vi "6612-00.vi"(8 "error in":errorcluster caption="错误输入") -> (0 "error out":errorcluster caption="错误输出", 3 "task out":refnum<k21> caption="任务输出")   [LabVIEW 2020]
uses:
  <vilib>/DAQmx/create/channels.llb/DAQmx Create Channel (CI-Position-Angular Encoder).vi
  <resource>/objmgr/daqmx.rc
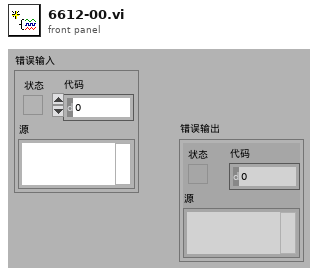
[diagram p1: front panel]
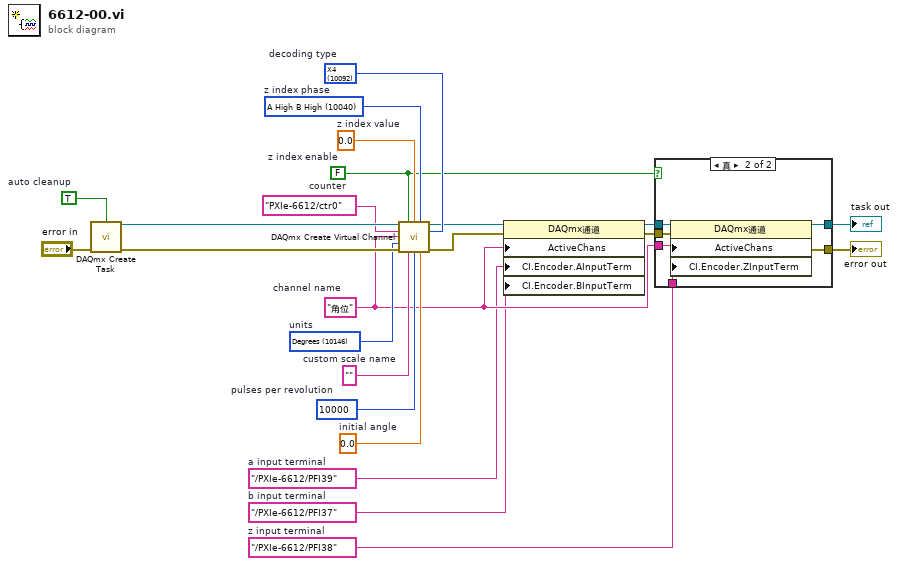
[diagram p0: block diagram]
diagram:
  w1 = "/PXIe-6612/PFI38"  # z input terminal
  w2 = "/PXIe-6612/PFI37"  # b input terminal
  w3 = "/PXIe-6612/PFI39"  # a input terminal
  w15 = 10146 items=["Degrees"=10146, "Radians"=10273, "Ticks"=10304, "From Custom Scale"=10065]  # units
  w11 = 10092 items=["X1"=10090, "X2"=10091, "X4"=10092, "Two Pulse Counting"=10313]  # decoding type
  w12 = 0.0  # initial angle
  w13 = u32 10000  # pulses per revolution
  w14 = ""  # custom scale name
  w16 = 10040 items=["A High B High"=10040, "A High B Low"=10041, "A Low B High"=10042, "A Low B Low"=10043]  # z index phase
  w17 = 0.0  # z index value
  w5 = FALSE  # z index enable
  w4 = "角位"  # channel name
  w19 = "PXIe-6612/ctr0"  # counter
  w21 = TRUE  # auto cleanup
  n1 = call <vilib>:"DAQmx Create Task.vi"("auto cleanup"=w21, "error in"="error in") -> ("task out"=w20:refnum<k21>, "error out"=w22:errorcluster)  [unwired: 12 in]
  n2 = call-poly <vilib>:"DAQmx Create Virtual Channel.vi"("task in"=w20, "z index enable"=w5, "z index value"=w17, "z index phase"=w16, "counter"=w19, "decoding type"=w11, "name to assign"=w4, "units"=w15, "error in"=w22, "custom scale name"=w14, "pulses per revolution"=w13, "initial angle"=w12) -> ("task out"=w10:refnum<k21>, "error out"=w18:errorcluster)  [unwired: 2 in]
  n3 = property class="DAQmx通道"(reference=w10, error in=w18, "ActiveChans"=w4, "CI.Encoder.AInputTerm"=w3, "CI.Encoder.BInputTerm"=w2) -> (reference out=w9:refnum<k21>, error out=w8:errorcluster)
  n4 = case "条件结构" shown="真" w5 {
    tunnel: w9 -> [w25 w31]
    tunnel: w8 -> [w24 w30]
    tunnel: [w25 w29] -> w7
    tunnel: [w24 w28] -> w6
    tunnel: w4 -> [_ w27]
    tunnel: w1 -> [_ w26]
    frame False {
    }
    frame True {
      n5 = property class="DAQmx通道"(reference=w31, error in=w30, "ActiveChans"=w27, "CI.Encoder.ZInputTerm"=w26) -> (reference out=w29:refnum<k21>, error out=w28:errorcluster)
    }
  }
  "error out" <- w6
  "task out" <- w7
